vi "Write FIFO.vi"(1 "Input Valid":bool, 2 "time":refnum<k21>, 3 "element":u64) -> (0 "ready for input":bool)   [LabVIEW 2021]
doc: "Writes data to two 32-bit FIFOs. This VI is a wrapper around the LabVIEW FPGA FIFO Write method. This VI exposes handshaking signals that inform the user when the FIFOs are ready to accept new data.\n\n<B>Input Parameters</B>\n\n<B>data in</B> is the data to be written to the FIFO.\n\n<B>enabled</B> specifies which streams are enabled.\n\n<B>input valid</B> specifies when 'data in' is valid.\n\n<B>reset</B> the LabVIEW FPGA FIFO.\n\n<B>fifo 0</B> is the reference to the FIFO to which data received on channel 0 will be written to.\n\n<B>fifo 1</B> is the reference to the FIFO to which data received on channel 1 will be written to.\n\n<B>Output Parameters</B>\n\n<B>ready for input</B> is a flow control signal that indicates whether the Write FIFO VI is ready to accept new data."
uses:
  <vilib>/rvi/DataTransferAndStorage/Container/Common/niFpgaContainerExecOnDevCompGetState.vi
  <vilib>/rvi/Emulation/niFpgaEmulationIsFPGAContextNoSignature.vi
  <vilib>/rvi/DataTransferAndStorage/Container/Common/niFpgaContainerGetUniqueNameForEmu.vi
  <vilib>/rvi/Memory/Memory_Emulation/niFpgaMemoryEmulationCacheClearOnFirstRun.vi
  <vilib>/rvi/Memory/Memory_Emulation/nirvimemoryEmulationManagerCache_MakeExclusive.vi
  <vilib>/rvi/Memory/Memory_Emulation/niFpgaMemoryEmulationValidateCache.vi
  <vilib>/rvi/Memory/Memory_Emulation/nirvimemoryEmulationManagerCache_InsertValue.vi
  <vilib>/Utility/error.llb/Clear Errors.vi
  <vilib>/rvi/Memory/Memory_Emulation/nirvimemoryEmulationManagerCache_ReleaseExclusive.vi
  <vilib>/rvi/Memory/Memory_Emulation/nirvimemoryEmulationManagerCache_GetValue.vi
  <vilib>/rvi/Memory/Memory_Emulation/nirvimemoryEmulationManagerCache_SetValue.vi
  <vilib>/rvi/Emulation/niFpgaProcessEmulError.vi
  <vilib>/rvi/Emulation/niFpgaSctlEmulationGetInTimedLoop.vi
  <vilib>/rvi/interface/RandomDataEmulation/nirviRandomDataMultiElementFPGAFIFO.vi
  <instcachedir>/0/nirviRandomDataMultiElementFPGAFIFO_3E9965BA1FAD4E7B8DABA31768A09B1F.lvgen/nirviRandomDataMultiElementFPGAFIFO_3E9965BA1FAD4E7B8DABA31768A09B1F_001.vi
  <vilib>/rvi/interface/RandomDataEmulation/niFpgaRandomDataHandleErrors.vi
  <vilib>/rvi/DataTransferAndStorage/Container/XNode/niFpgaContainer.xnode
  <vilib>/rvi/DataTransferAndStorage/Register/Emulation/niFpgaRegisterEmulationRefIn.vi
  <vilib>/rvi/interface/RandomDataEmulation/nirviRandomDataFpgaMultiElementTemplate.vi
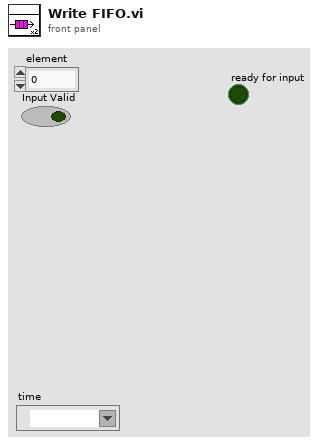
[diagram p1: front panel]
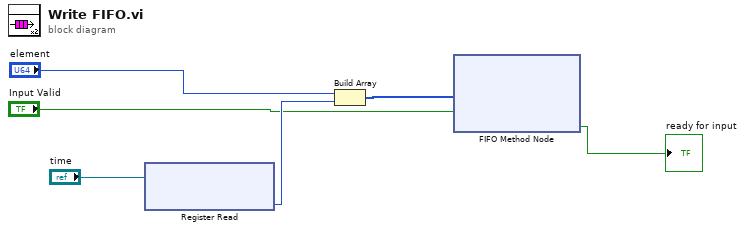
[diagram p0: block diagram]
diagram:
  n1 = xnode "Register Read"("Register In"="time") -> ("Data"=w5:u64)  [unwired: 1 out]
  n2 = Build Array("element", w5) -> (w4:u64[])
  n3 = xnode ("FIFO Method Node")("Element"=w4, "Input Valid"="Input Valid") -> ("Ready for Input"=→"ready for input":bool)  [unwired: 1 in, 1 out]
